vi "ControlsAndIndicators.vi"() -> ()   [LabVIEW 2019]
panel:
  out "Meter":dbl(knob) scale=0.0..10.0
  in  "Knob":dbl(knob) scale=0.0..10.0
  out "Thermometer":dbl(slide) scale=0.0..100.0
  in  "Slide":dbl(slide) scale=0.0..10.0
  out "Boolean":bool
  in  "Numeric":dbl
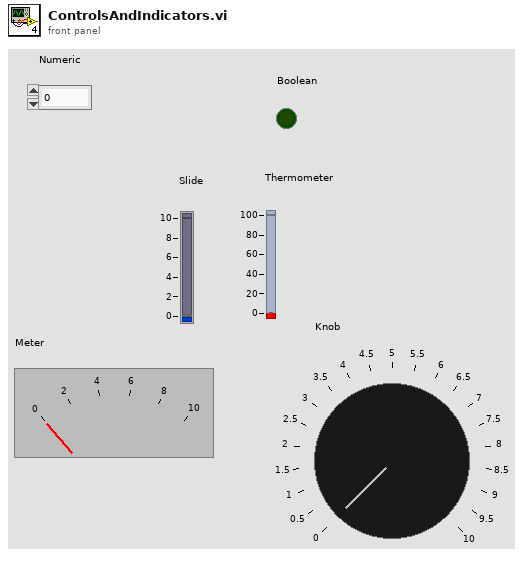
[diagram p1: front panel]
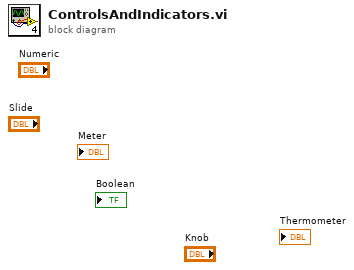
[diagram p0: block diagram]
diagram:
